vi "FTW-ActorExtended-Ask.vi"(0 "FTW-ActorExtended In":refnum<class "FTW-ActorExtended.lvclass">, 5 "Publisher Name":string, 7 "Message Header":string, 9 "Message Body":string, 11 "error in":errorcluster) -> (4 "FTW-ActorExtended Out":refnum<class "FTW-ActorExtended.lvclass">, 6 "Response Header":string, 8 "Response Body":string, 10 "Timed out?":bool, 14 "Roundtrip Time":dbl format="%.6fsec", 15 "error out":errorcluster)   [LabVIEW 2013, in "FTW-ActorExtended.lvclass"]
uses:
  FTW-ActorExtended.lvclass
  FTW-ActorExtended.lvclass/FTW-ActorExtended.ctl
  Connector/FTW-ActorConnector.lvclass
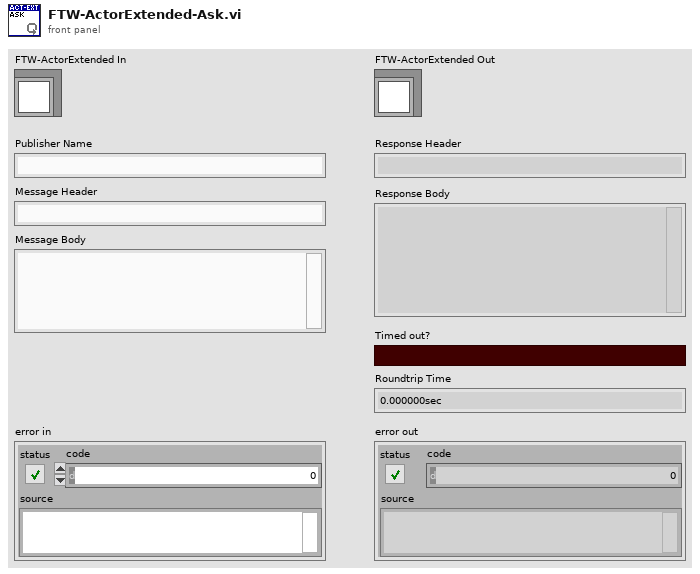
[diagram p1: front panel]
types:
  T1 = cluster{"Name":string, "URI":string, "Connector":refnum<class "FTW-ActorConnector.lvclass">}[]
  T2 = cluster{"Name":string, "URI":string, "Connector":refnum<class "FTW-ActorConnector.lvclass">}
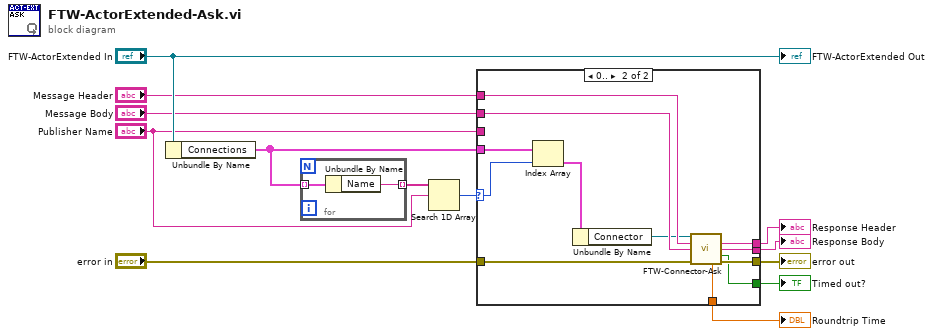
[diagram p0: block diagram]
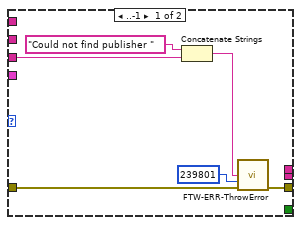
[diagram p2: hidden frame]
diagram:
  n1 = Unbundle By Name("FTW-ActorExtended In") -> ("Connections"=w11:T1)
  n2 = for {
    tunnel: w11 -> [w15] mode=indexing
    tunnel: [w14] -> w1 mode=indexing
    n3 = Unbundle By Name(w15) -> ("Name"=w14:string)
  }
  n4 = Search 1D Array(1D array=w1, element="Publisher Name") -> (index of element=w12:i32)  [unwired: 1 in]
  n5 = case shown="0.." w12 {
    selector: w12 -> [_ w33]
    tunnel: w11 -> [_ w32]
    tunnel: [w20 w30] -> w10
    tunnel: "error in" -> [w21 w31]
    tunnel: "Publisher Name" -> [w16 _]
    tunnel: "Message Header" -> [_ w29]
    tunnel: "Message Body" -> [_ w28]
    tunnel: [_ w27] -> w5
    tunnel: [_ w26] -> w4
    tunnel: [_ w25] -> w3
    tunnel: [_ w24] -> w2
    frame ..-1 {
      n6 = Concatenate Strings("Could not find publisher " ("Error Message"), w16) -> (w17:string)
      n7 = call "FTW-ERR-ThrowError.vi"("Error Message"=w17, "Error Code"=239801, "error in"=w21) -> ("error out"=w20:errorcluster)  [unwired: 12 in]
    }
    frame 0.. {
      n8 = Index Array(array=w32, index=w33) -> (element=w23:T2)
      n9 = Unbundle By Name(w23) -> ("Connector"=w22:refnum<class "FTW-ActorConnector.lvclass">)
      n10 = call "FTW-Connector-Ask.vi"("FTW Actor Connector"=w22, "Request Header"=w29, "Request Body"=w28, "error in"=w31) -> ("Response Header"=w24:string, "Response Body"=w25:string, "Timed out?"=w26:bool, "Roundtrip Time"=w27:dbl, "error out"=w30:errorcluster)  [unwired: 6 in, 1 out]
    }
  }
  "error out" <- w10
  "Timed out?" <- w4
  "Response Header" <- w2
  "Response Body" <- w3
  "Roundtrip Time" <- w5
  "FTW-ActorExtended Out" <- "FTW-ActorExtended In"
